vi "IMUOrientOpen.vi"(0 "Op Mode":T6(ring)=enum."NDOF", 1 "Calibrate?":bool, 3 "Stored Cal File":string="BNO055 Cal MC P3 11-28-2015 145653", 5 "Placement":T8(ring)=enum."P3", 9 "I2C Bus":T3=enum."I2C MXP", 11 "Status delay":i32=30, 12 "Alt Adr?":bool, 14 "Flash?":bool) -> (2 "Occupant":u8[](array[numeric]) format="%02x", 4 "IMU Dev Ref":T1={"I2CDevRef"={"DevStatus"={"status"=FALSE, "code"=0, "source"=""}, "Device Address"=0, "Handle"=0, "I2C Bus"=enum."Invalid"}, "Valid Cal File?"=FALSE} {"I2CDevRef"."Device Address" format="%.0x"}, 6 "Cal Status @ Open":T4, 8 "error out":errorcluster, 10 "Fatal Result":bool, 13 "Odd":bool, 15 "Bad Result":bool)   [LabVIEW 2017]
uses:
  <vilib>/Rock Robotics/SystemInterfaces/i2clib/i2c_bus.ctl
  <userlib>/836-Library/Sensor/IMU/Setup State.ctl
  <userlib>/836-Library/Sensor/IMU/ImuDevRef.ctl
  <vilib>/Rock Robotics/WPI/I2C/WPI_I2CDevRef.ctl
panel:
  out "Adr":u8 format="%02x"
  out "Restore Cal ct":i32
  out "Bad ct":i32
  out "SC ct":i32
  out "S":T5
  out "G":T5
  out "A":T5
  out "M":T5
  out "Bad Result":bool
  out "Fusion":bool
  out "Fusion ct":i32
  out "Reset ct":i32
  out "Setup ct":i32
  out "Setup State":T7
  # "Manual Cal\nCalibration Status Indicator"
  # "Diagnostics"
  # "These controls/indicators are non-operational / they are here as example documentation only."
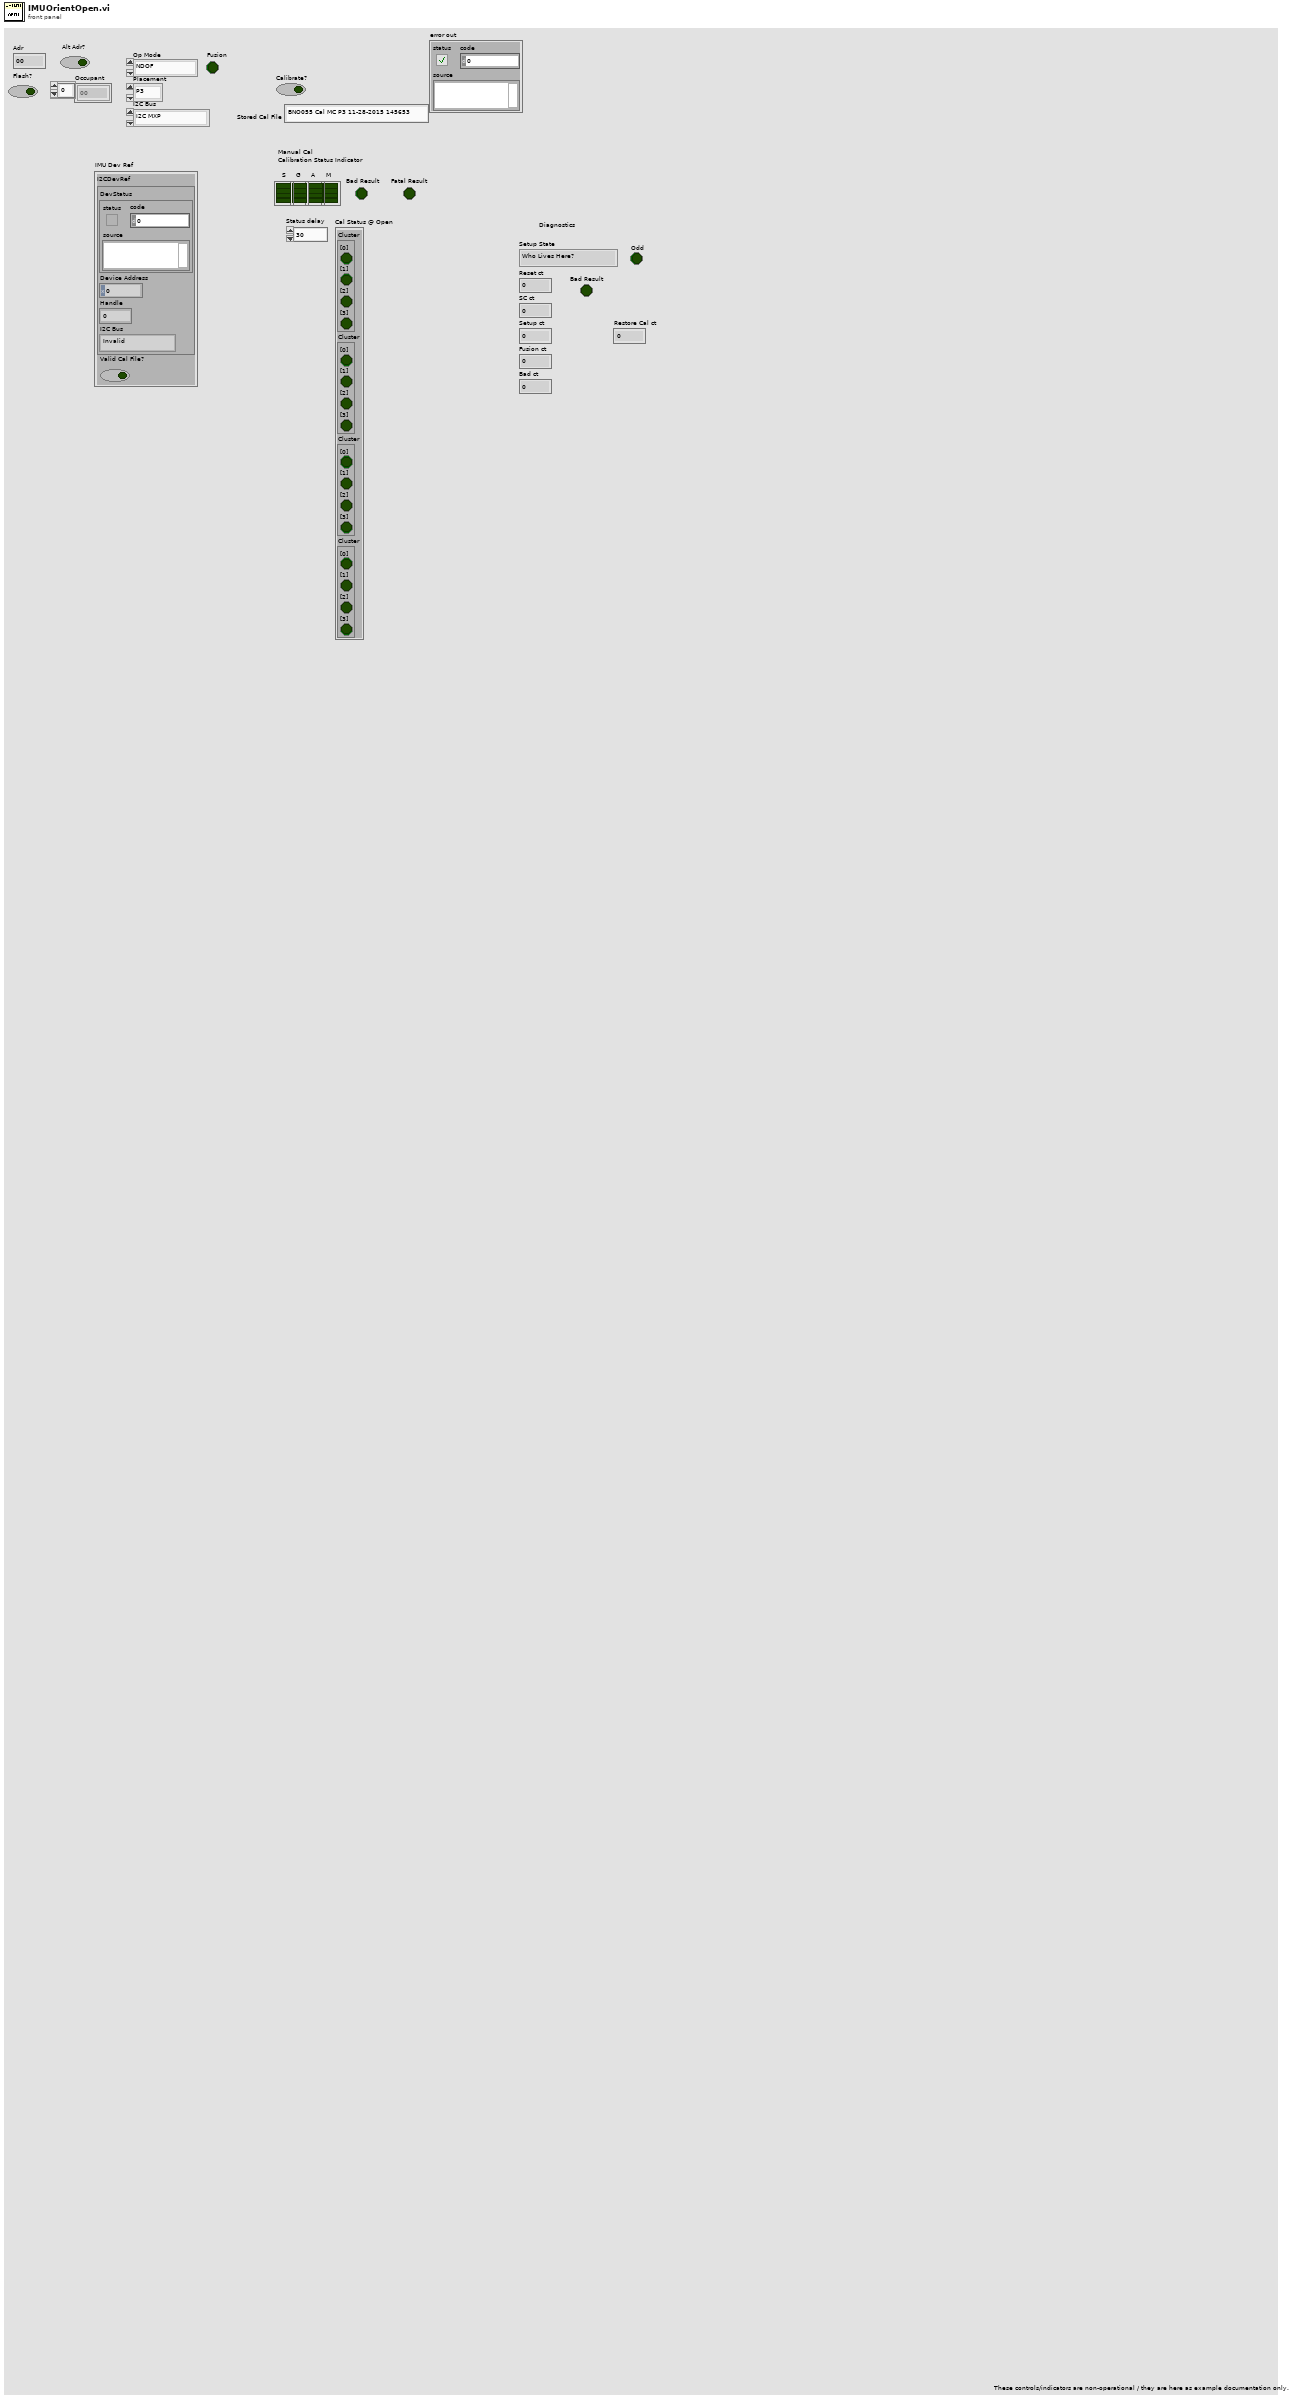
[diagram p1: front panel]
types:
  T1 = typedef "ImuDevRef.ctl" = cluster{"I2CDevRef":T2, "Valid Cal File?":bool}
  T2 = typedef "WPI_I2CDevRef.ctl" = cluster{"DevStatus":errorcluster, "Device Address":u8, "Handle":i32, "I2C Bus":T3}
  T3 = typedef "i2c_bus.ctl" = enum16{"I2C On-Board", "I2C MXP", "Invalid"}
  T4 = cluster{"Cluster":cluster{"[0]":bool, "[1]":bool, "[2]":bool, "[3]":bool}, "Cluster":cluster{"[0]":bool, "[1]":bool, "[2]":bool, "[3]":bool}, "Cluster":cluster{"[0]":bool, "[1]":bool, "[2]":bool, "[3]":bool}, "Cluster":cluster{"[0]":bool, "[1]":bool, "[2]":bool, "[3]":bool}}
  T5 = cluster{"Boolean":bool, "Boolean 2":bool, "Boolean 3":bool, "Boolean 4":bool}
  T6 = enum8{"ConfigMode", "AccOnly", "MagOnly", "GyroOnly", "AccMag", "AccGyro", "MagGyro", "AMG", "IMU", "Compass", "M4G", "NDOF_FMC_OFF", "NDOF"}
  T7 = typedef "Setup State.ctl" = enum16{"Who Lives Here?", "Config Mode", "Page 0", "Reset", "Units, Xtal, & Placement", "Fusion Mode", "Pre Calibration", "Error Check", "Manual Cal", "Save Cal", "Restore Cal", "Cal Status", "Idle"}
  T8 = enum32{"P0", "P1", "P2", "P3", "P4", "P5", "P6", "P7"}
  T9 = enum16{"open", "open or create", "create or replace", "create", "open (read-only)"}
  T10 = enum8{"ConfigMode", "AccOnly", "MagOnly", "GyroOnly", "AccMag", "AccGyro", "MagGyro", "AMG", "IMU", "Compass", "M4G", "NDOF_FMC_OFF", "NDOF"}[]
  T11 = cluster{"[0]":bool, "[1]":bool, "[2]":bool, "[3]":bool}
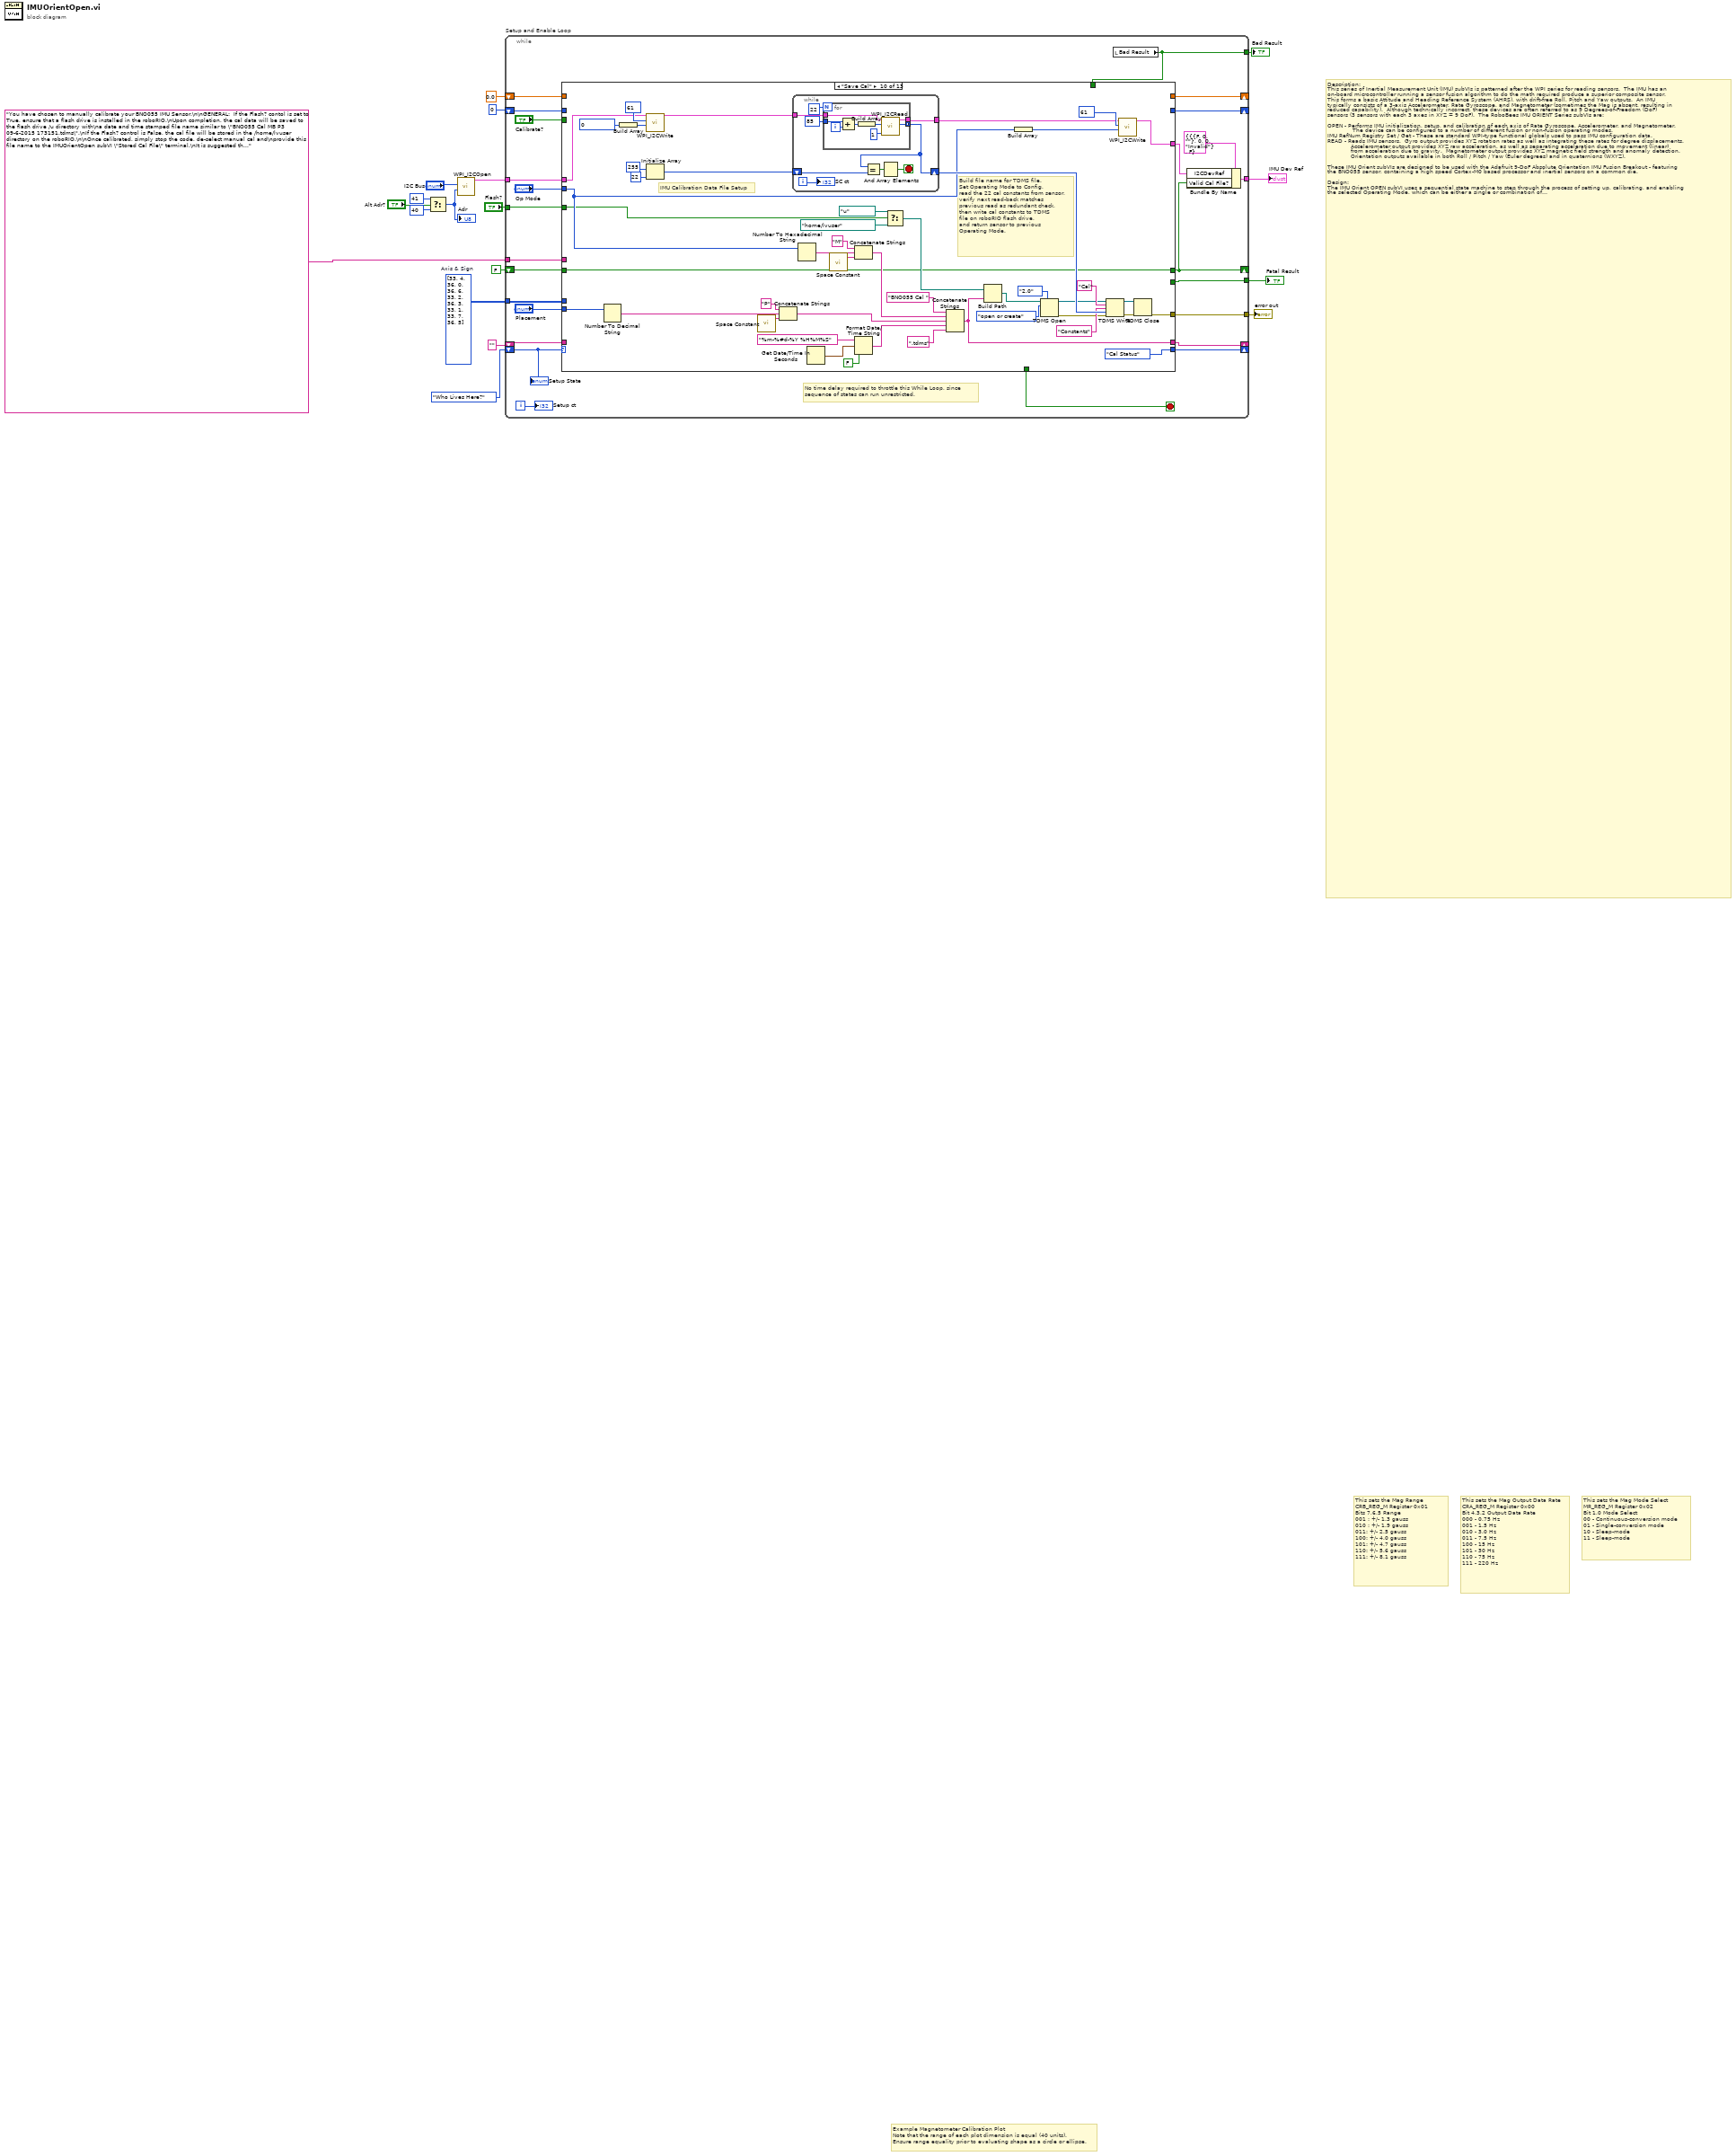
[diagram p0: block diagram]
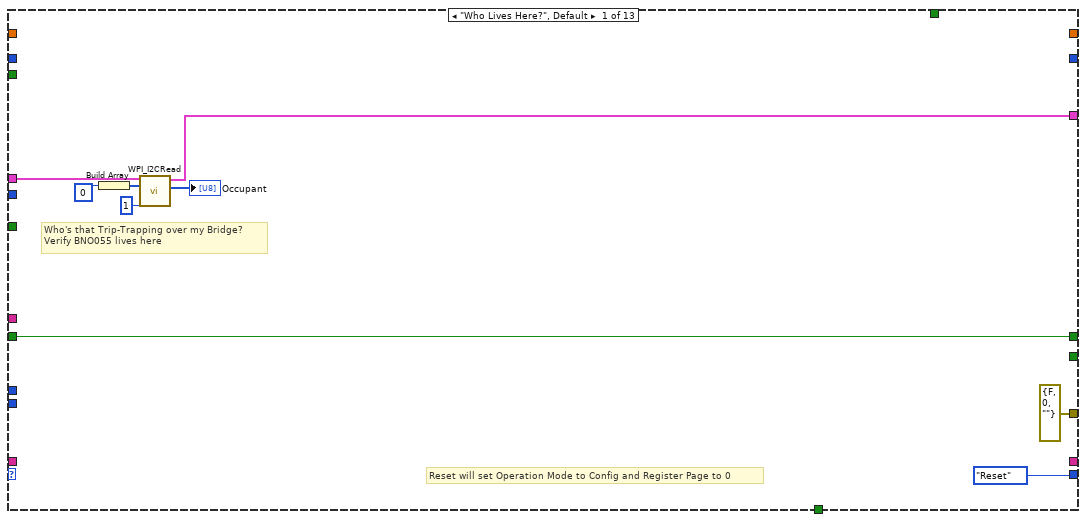
[diagram p2: hidden frame]
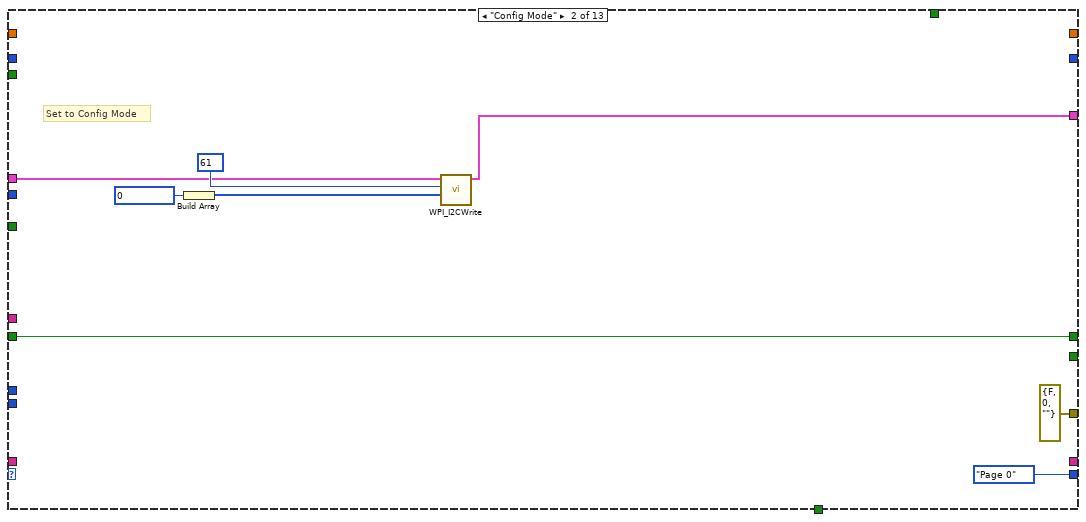
[diagram p3: hidden frame]
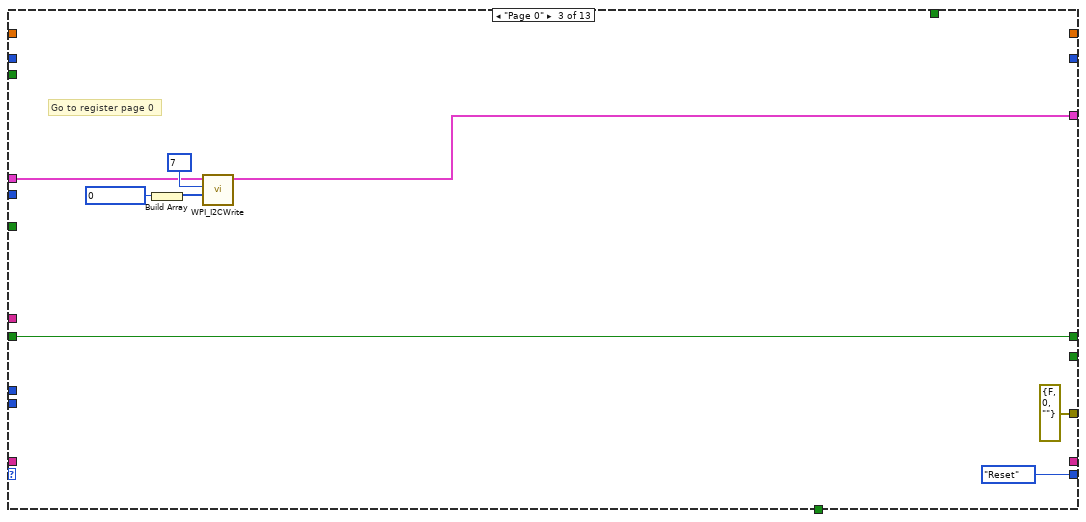
[diagram p4: hidden frame]
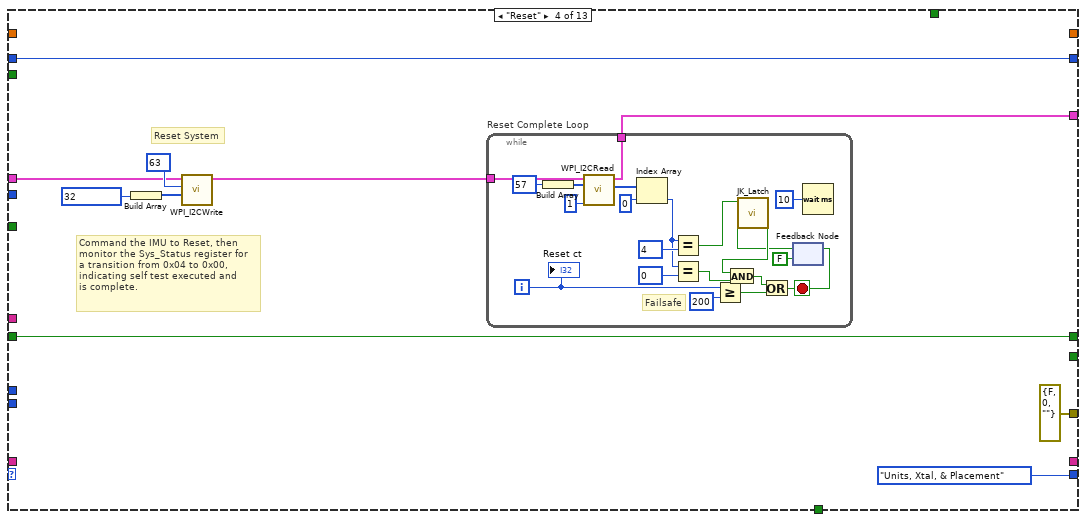
[diagram p5: hidden frame]
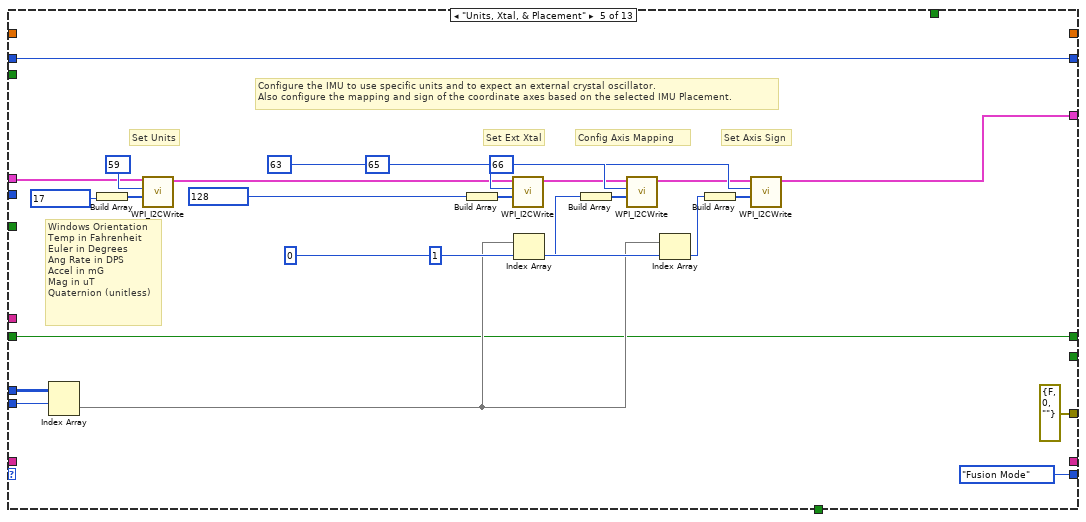
[diagram p6: hidden frame]
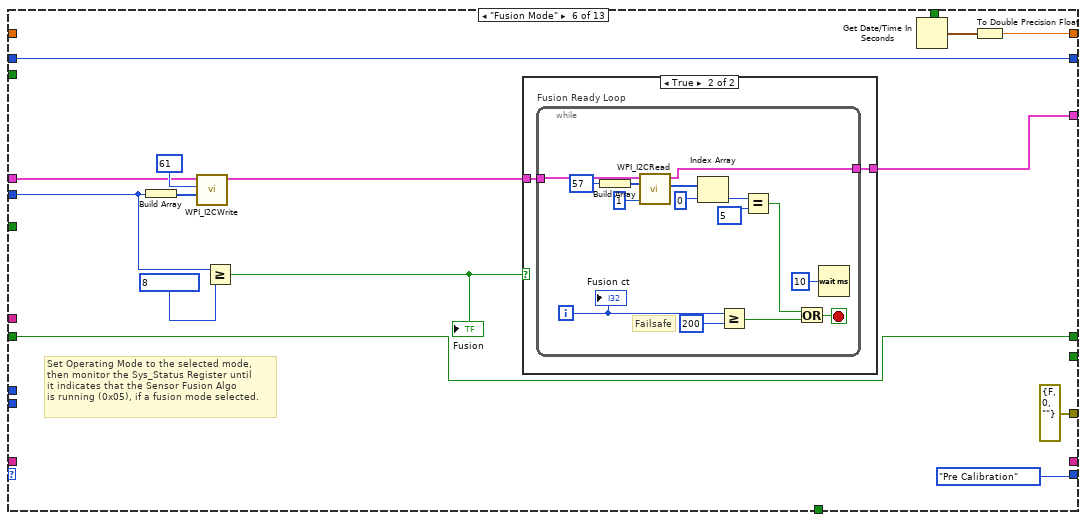
[diagram p7: hidden frame]
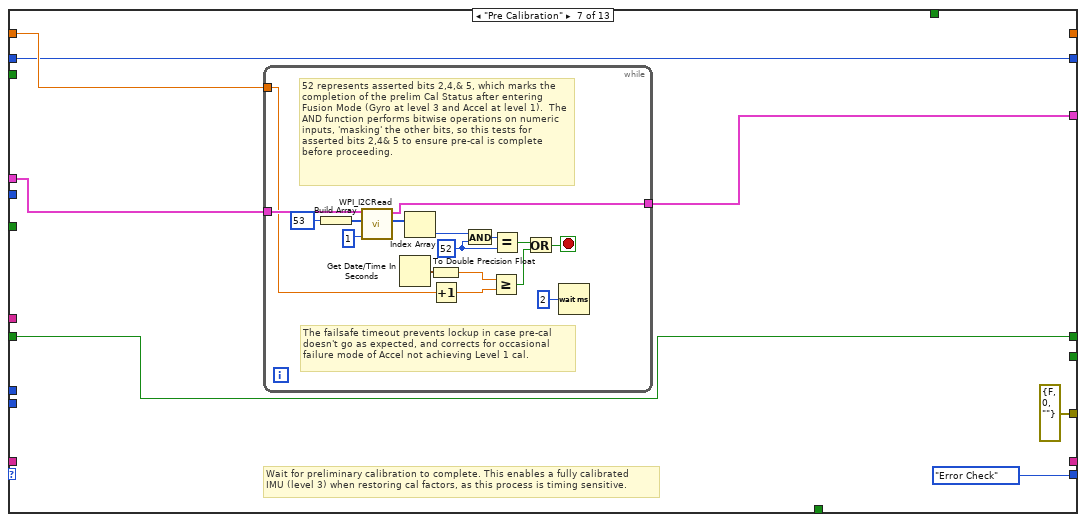
[diagram p9: hidden frame]
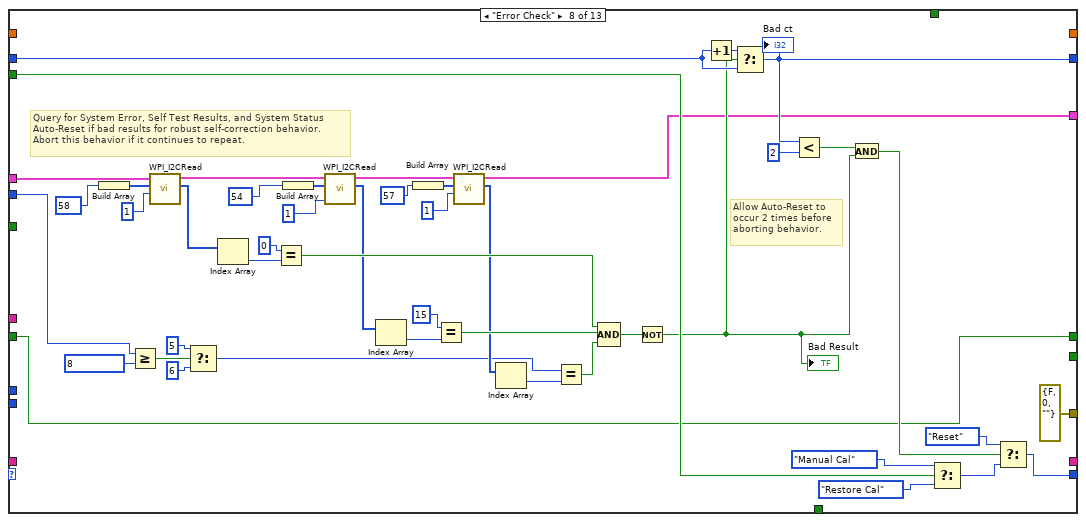
[diagram p10: hidden frame]
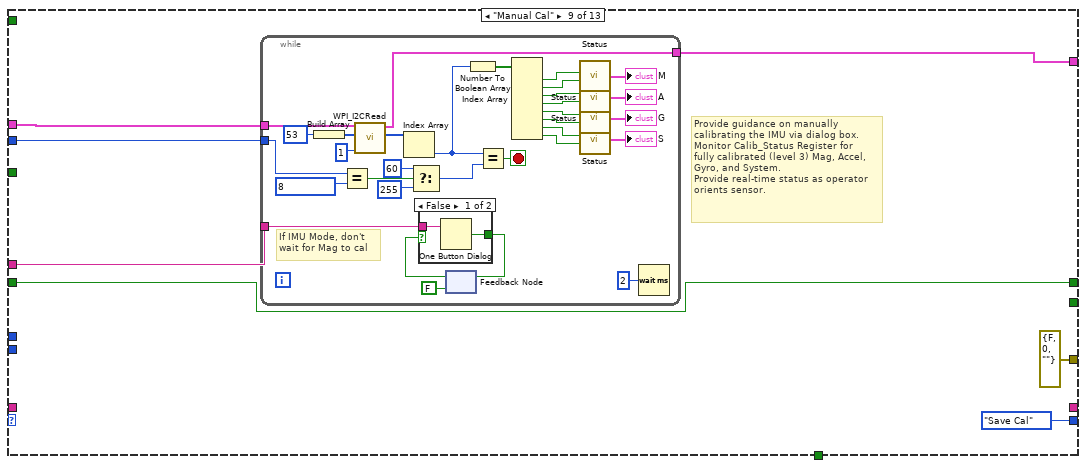
[diagram p11: hidden frame]
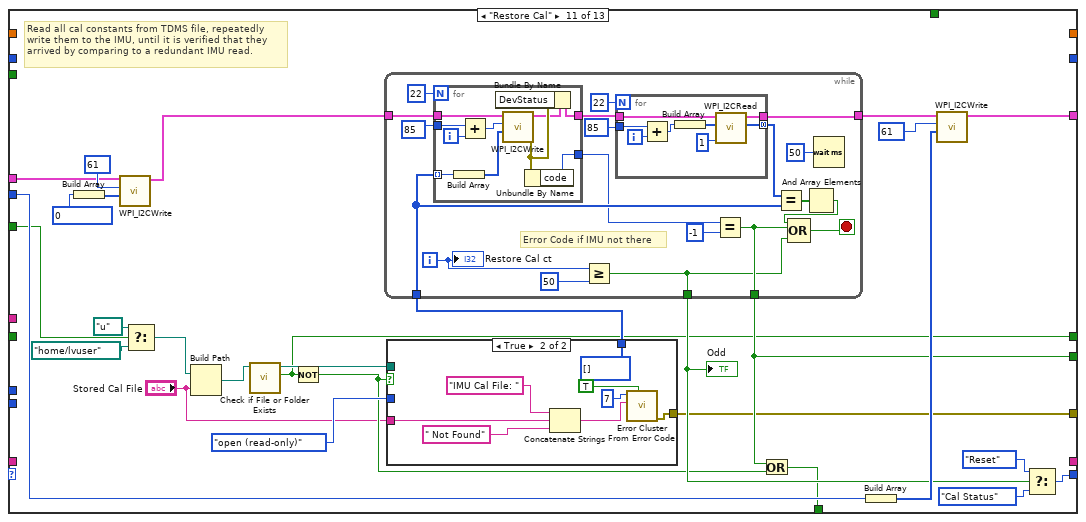
[diagram p13: hidden frame]
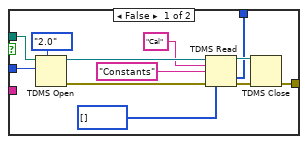
[diagram p14: hidden frame]
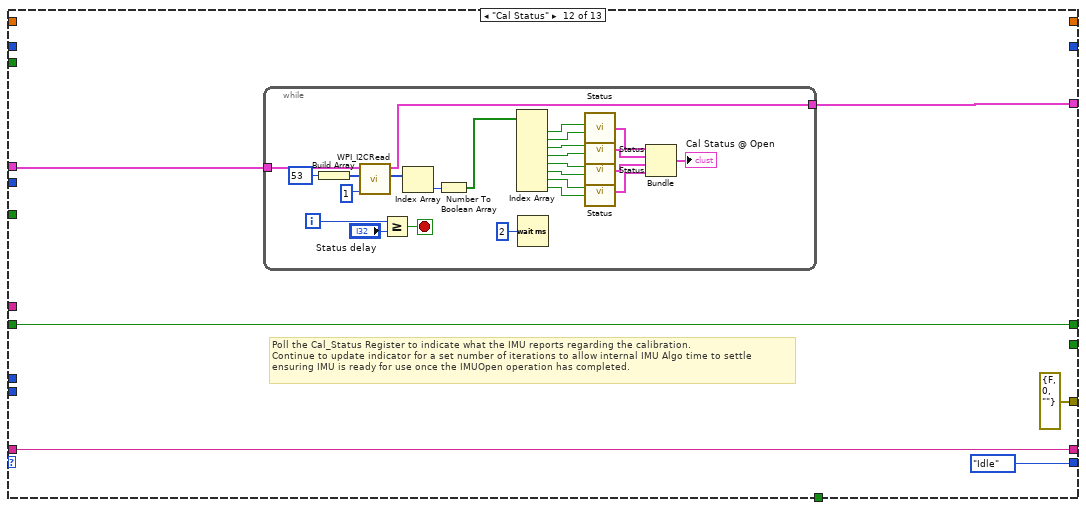
[diagram p15: hidden frame]
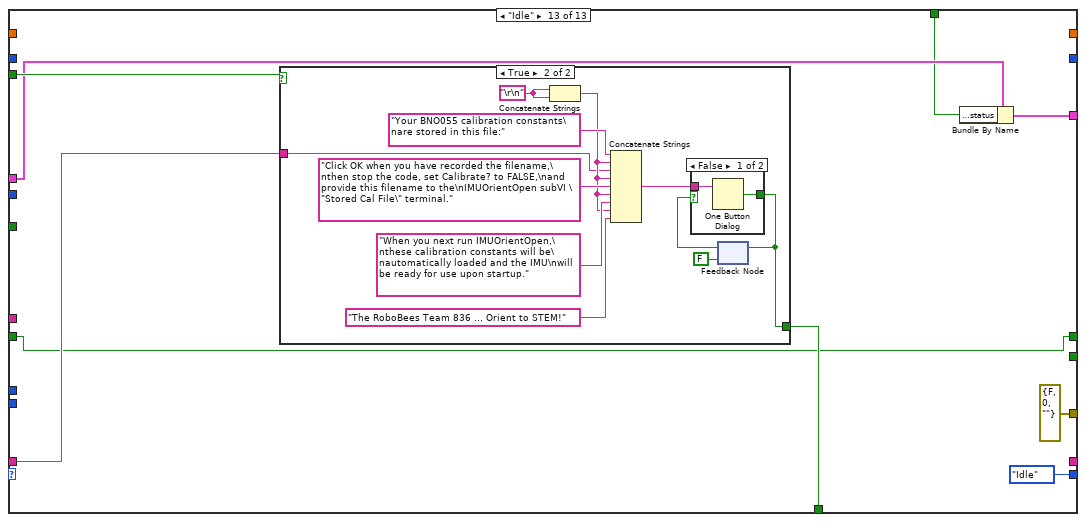
[diagram p16: hidden frame]
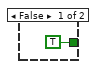
[diagram p17: hidden frame]
diagram:
  w15 = u8[][] [[33, 4], [36, 0], [36, 6], [33, 2], [36, 3], [33, 1], [33, 7], [36, 5]]  # Axis & Sign
  # "Description:\nThis series of Inertial Measurement Unit (IMU) subVIs is patterned after the WPI series for reading sensors.  The IMU has an\non-board microcontroller running a sensor fusion algorithm to do the math required produce a superior composite sensor.\nThis forms a basic Attitude and Heading Reference System (AHRS), with drift-free Roll, Pitch and Yaw outputs.  An IMU\ntypically consists of a 3-axis Accelerometer, Rate Gyroscope, and Magnetometer (sometimes the Mag is absent, resulting in\nreduced capability).  Although technically incorrect, these devices are often referred to as 9 Degrees-of-Freedom (DoF)\nsensors (3 sensors with each 3 axes in XYZ = 9 DoF).  The RoboBees IMU ORIENT Series subVIs are:\n\nOPEN - Performs IMU initialization, setup, and calibration of each axis of Rate Gyroscope, Accelerometer, and Magnetometer.\n              The device can be configured to a number of different fusion or non-fusion operating modes.\nIMU RefNum Registry Set / Get - These are standard WPI-type functional globals used to pass IMU configuration data.\nREAD - Reads IMU sensors.  Gyro output provides XYZ rotation rates as well as integrating these rates for degree displacements.\n             Accelerometer output provides XYZ raw acceleration, as well as separating acceleration due to movement (linear)\n             from acceleration due to gravity.  Magnetometer output provides XYZ magnetic field strength and anomaly detection.\n             Orientation outputs available in both Roll / Pitch / Yaw (Euler degrees) and in quaternions (WXYZ).\n\nThese IMU Orient subVIs are designed to be used with the Adafruit 9-DoF Absolute Orientation IMU Fusion Breakout - featuring\nthe BNO055 sensor, containing a high speed Cortex-M0 based processor and inertial sensors on a common die.\n\nDesign:\nThe IMU Orient OPEN subVI uses a sequential state machine to step through the process of setting up, calibrating, and enabling\nthe selected Operating Mode, which can be either a single or combination of sensors running in a non-fusion mode, or one of\nseveral fusion operating modes.\n\nThe IMU breakout board from Adafruit.com has a single I2C bus for communication.  The sensor I2C Address (in hex) and\ndata sheet for I2C register references are:\n\nI2C Address  -  Data Sheet Reference -\thttps://ae-bst.resource.bosch.com/media/_tech/media/datasheets/BST_BNO055_DS000_14.pdf\n       0x28        -  (Main I2C address, used when Alt Adr? control is False)\n       0x29        -  (Alternate I2C address is used when Alt Adr? control is asserted or True)\n\nNote: The Adafruit website links to an older version of the BNO055 spec sheet (ver 1.2).  The Bosch site will maintain the latest\nversion.  The link above is the latest revision (ver 1.4) as of January 2017 (released June 2016).   This is a highly sophisticated\nsensor, with many control options, so it is recommended that one review the spec sheet to understand all its capabilities.\n\nSome design effort was expended in an attempt to ensure high reliability of operation.  Data transfer between the sensor cal registers\nand the cal file storage location (RIO or flash drive, where cal constants are stored during power down periods) is redundantly verified\nto be successful.  (Testing indicated this to be necessary.)  Upon initialization, if the sensor fails its internal self test, the code will\nattempt to reset the sensor.  This will only occur two times to avoid an infinite loop, which might otherwise prevent a robot from\nexecuting operations code.\n\nCalibration:\nRaw readings from an IMU are not very useful until they are conditioned by carefully determined calibration parameters.  One of\nthe key differences between this IMU and others, such as the one discussed here: \n\n                                                         http://www.chiefdelphi.com/forums/showthread.php?t=131823 \n\nis that this BNO055 contains an integrated microcontroller, running a sensor fusion algorithm, which is designed to constantly\nself-calibrate in real-time, after an initial calibration process has occurred.  So, unlike other IMUs that require interface code, this\nIMU really only requires code to trigger the on-board calibration code.  This makes the code for the sensor READ operations simple,\nand the complex code integration requirement associated only with the sensor OPEN (although one only has to trigger the on-board\ncal process, doing this reliably and providing functionality to store/reload the results still drives code sophistication requirements).\n\nOnce the state machine has initialized the sensor, a user-selected control is referenced to either initiate the sensor's embedded\ncal process or read previously stored calibration constants from a file.  [Note: this vi expects a flash drive to be installed in one\nof the roboRIOs USB ports for cal file storage/retrieval, if the Flash? control is asserted].   A dialog box is used to instruct the user\non the sensor movements required for calibration, and a Calibration Status Indicator is provided on this vi's front panel to provide\nfeedback and track progress.   Once cal is complete, the filename containing the cal constants is displayed.  De-selecting the cal\ncontrol and providing the cal filename to this vi enables the sensor to open in a ready-for-use state.\n\nThe cal filename will contain the Operating Mode, Placement (sensor orientation), and a timestamp to help distinguish one file\nfrom another.  The Op Mode and Placement are included as there is some indication in testing that one should not expect the cal\nto be correct when these parameters differ between cal and use.\n\nVI Properties:\nExecution Reentrancy is set to Pre Allocated Clone Reentrant Execution, enabling multiple Open instances for mutiple IMUs\n\nImplementation:\nIt is recommended that the MXP I2C Interface is used, rather than the On-Board I2C Interface, as the latter can generate glitches from\nLo/Hi byte pairing failures when data is reassembled across paired measurement registers.\n\nA visualization vi is provided to observe orientation change as the sensor is moved.  The vi runs on the My Computer Target,\n(not the roboRIO Target), which means it can only be accessed in debug mode.  There is an issue where Roll exceeding ~45 degrees\ncauses an orientation error.\n \nIt is important to note that while the P/R/Y values are constrained, the Gyro displacement values in X/Y/Z are not.  Gyro deg outputs\nfrom the IMU ORIENT READ subVI will wind (not wrap) - i.e. they will continue to count above/below 360 degrees.  Use the LabVIEW\nQuotient & Remainder (modulus) function to convert these outputs to a wrapping behavior, if desired. \n\nImplementation considerations for IMU Read:\nThis design performs numerical integration off-FPGA for the Digital Gyro (unlike the Analog Gyro subVIs, which typically utilize\nthe FPGA to perform accumulation for superior speed resulting in less integration error).   Testing indicates this off-FPGA\napproach may be adequate for FRC application, however, it is important to ensure the code runs without any timing issues.\nThis is why a Timed Loop is recommended for the IMU Read within Periodic Tasks (executes at a higher priority).  Non-uniformity\nin read iteration is mitigated by design, as each dt is uniquely calculated by time stamping each read event.  This means that while\nsome variation in timing can be tolerated (the occasional late iteration), excessively long durations (periods) between successive\nreads will fail to capture the actual rate profile as it changes resulting in integration error.  \n\nIn short, use a Timed Loop structure to iterate IMU READs, and set the loop period for a relatively fast iteration (<75 ms).  Shorter\nperiods provide improved accuracy of degree displacements, however setting this too short can impact the execution of your\nremaining code (especially when using Timed Loops).  One way of determining an optimized period is to set it while monitoring\nthe \"Finished Late?\" Loop parameter, ensuring this value stays False.   It helps if the CPU Utilization remains low (<75%), which\ncan be monitored with the RT Get CPU Loads subVI (Real Time menu).  Study LabVIEW determinism for additional insight.\n\n----- RoboBees FRC Team 836! -----  You too can conquer inertia!! ... ORIENT on a career in STEM!"
  # "Example Magnetometer Calibration Plot\nNote that the range of each plot dimension is equal (40 units).\nEnsure range equality prior to evaluating shape as a circle or ellipse."
  # "This sets the Mag Mode Select\nMR_REG_M Register 0x02\nBit 1,0 Mode Select\n00 - Continuous-conversion mode \n01 - Single-conversion mode\n10 - Sleep-mode\n11 - Sleep-mode"
  # "This sets the Mag Output Data Rate\nCRA_REG_M Register 0x00\nBit 4,3,2 Output Data Rate\n000 - 0.75 Hz \n001 - 1.5 Hz \n010 - 3.0 Hz\n011 - 7.5 Hz\n100 - 15 Hz\n101 - 30 Hz\n110 - 75 Hz\n111 - 220 Hz"
  # "This sets the Mag Range\nCRB_REG_M Register 0x01\nBits 7,6,5 Range\n001 : +/- 1.3 gauss\n010 : +/- 1.9 gauss\n011: +/- 2.5 gauss\n100: +/- 4.0 gauss\n101: +/- 4.7 gauss\n110: +/- 5.6 gauss\n111: +/- 8.1 gauss"
  n1 = Select(t=u8 41 ("Device Address"), s="Alt Adr?", f=u8 40 ("Device Address")) -> (s? t:f=w6:u8)
  "Adr" <- w6
  n2 = call <vilib>:"WPI_I2COpen.vi"("Device Address"=w6, "I2C Bus"="I2C Bus") -> ("I2CDevRef"=w16:T2)  [unwired: 8 in, 1 out]
  n3 = while "Setup and Enable Loop" {
    tunnel: w16 -> [w37]
    tunnel: "You have chosen to manually calibrate your BNO055 IMU Sensor.\n\nGENERAL:  If the Flash? contol is set to True, ensure that a flash drive is installed in the roboRIO.\nUpon completion, the cal data will be saved to the flash drive /u directory with\na date and time stamped file name similar to \"BNO055 Cal MB P3 09-6-2015 173151.tdms\".\nIf the Flash? control is False, the cal file will be stored in the /home/lvuser directory on the roboRIO.\n\nOnce calibrated, simply stop the code, de-select manual cal and\nprovide this file name to the IMUOrientOpen subVI \"Stored Cal File\" terminal.\nIt is suggested that manual calibration be performed whenever one re-locates\nthe IMU sensor or adds/changes the metallic configuration of the robot.\n\nPREPARATIONS:  If sensor is installed on a robot, ensure sensor is secure.\nThese device movement instructions will then apply to entire robot.\nAs you proceed, monitor the Calibration Status Indicator on the IMUOrientOpen Front Panel.\nCalibration is complete when all indicators are Green.\n\nGYRO CAL:  Allow device to maintain a single stable\nposition to enable Gyro to self-calibrate.\n\nACCELEROMETER CAL:  Place device in 6 different stable\npositions for a few seconds to allow it to calibrate.\nEnsure there is slow movement between 2 stable positions.\nThe 6 stable positions can be in any direction, but ensure the\ndevice is perpendicular to the X,Y & Z axis at least once.\nThis is usually the most difficult device to calibrate.\nIf problematic, try slowing down the movement between positions.\n\nMAGNETOMETER CAL:  Make random movements\nin all 3 axes until Cal Status Indicator is Green.\n\nSYSTEM CAL:  Alternately move device and hold still until\nCal Status Indicator is Green, if necessary. \n\nClick OK when ready to begin." ("message") -> [w42]
    tunnel: w15 -> [w40]
    shift-right: [w35] -> _
    shift-left: 0 -> [w34]
    tunnel: [w26] -> w13
    shift-right: [w33] -> _
    shift-left: 0.0 -> [w32]
    shift-right: [w31] -> _
    shift-left: "" -> [w30]
    shift-right: [w29] -> _
    shift-left: Setup_State."Who Lives Here?" -> [w28]
    tunnel: [w27] -> w9
    tunnel: "Flash?" -> [w25]
    tunnel: [w24] -> w3
    tunnel: [w21] -> w2
    shift-right: [w20] -> _
    shift-left: FALSE ("file or folder exists?") -> [w19]
    i -> [w39]
    stop <- w38 stop-if-true
    # "No time delay required to throttle this While Loop, since sequence of states can run unrestricted."
    n4 = local read "Bad Result"() -> (w26:bool)
    n5 = case shown="\"Save Cal\"" w28 {
      tunnel: [Setup_State."Reset" Setup_State."Page 0" Setup_State."Reset" Setup_State."Units, Xtal, & Placement" Setup_State."Fusion Mode" Setup_State."Pre Calibration" Setup_State."Error Check" w200 Setup_State."Save Cal" Setup_State."Cal Status" w341 Setup_State."Idle" Setup_State."Idle"] -> w29
      tunnel: w37 -> [w49 w56 w65 w75 w117 w137 w164 w216 w234 w309 w354 w423 w453]
      tunnel: "Calibrate?" -> [_ _ _ _ _ _ _ w188 _ _ _ _ w457]
      tunnel: [_ _ _ _ _ w134 _ _ _ _ _ _ _] -> w33
      tunnel: w32 -> [_ _ _ _ _ _ w162 _ _ _ _ _ _]
      tunnel: w42 -> [_ _ _ _ _ _ _ _ w232 _ _ _ _]
      tunnel: "Placement" -> [_ _ _ _ w107 _ _ _ _ w283 _ _ _]
      tunnel: w40 -> [_ _ _ _ w105 _ _ _ _ _ _ _ _]
      tunnel: [_ _ _ _ _ _ _ _ _ w280 _ w421 _] -> w31
      tunnel: [_ _ _ _ _ _ _ _ _ _ w338 _ w456] -> w38
      tunnel: w30 -> [_ _ _ _ _ _ _ _ _ _ _ w421 w455]
      tunnel: "Op Mode" -> [_ _ _ _ _ w130 _ w193 w230 w279 w350 _ _]
      tunnel: [_ _ _ w72 w103 w129 w161 w190 _ _ _ _ _] -> w35
      tunnel: w34 -> [_ _ _ w72 w103 w129 w161 w191 _ _ _ _ _]
      tunnel: [_ _ _ _ _ _ _ _ _ _ w339 _ _] -> w27
      tunnel: [w46 w55 w63 w71 w102 w128 w160 w184 w231 w278 w349 w420 w452] -> w22
      tunnel: w26 -> [_ _ _ _ _ _ _ _ _ _ _ _ w451]
      tunnel: w25 -> [_ _ _ _ _ _ _ _ _ w274 w346 _ _]
      tunnel: [errorcluster {"status"=FALSE, "code"=0, "source"=""} ("error out") errorcluster {"status"=FALSE, "code"=0, "source"=""} ("error out") errorcluster {"status"=FALSE, "code"=0, "source"=""} ("error out") errorcluster {"status"=FALSE, "code"=0, "source"=""} ("error out") errorcluster {"status"=FALSE, "code"=0, "source"=""} ("error out") errorcluster {"status"=FALSE, "code"=0, "source"=""} ("error out") errorcluster {"status"=FALSE, "code"=0, "source"=""} ("error out") errorcluster {"status"=FALSE, "code"=0, "source"=""} ("error out") errorcluster {"status"=FALSE, "code"=0, "source"=""} ("error out") w273 w334 errorcluster {"status"=FALSE, "code"=0, "source"=""} ("error out") errorcluster {"status"=FALSE, "code"=0, "source"=""} ("error out")] -> w24
      tunnel: [w44 w53 w61 w69 w100 w126 w158 w182 w228 w270 w333 w418 w449] -> w20
      tunnel: w19 -> [w44 w53 w61 w69 w100 w126 w158 w182 w228 w270 _ w418 w449]
      frame "Who Lives Here?", Default {
        # "Reset will set Operation Mode to Config and Register Page to 0"
        # "Who's that Trip-Trapping over my Bridge?\nVerify BNO055 lives here"
        n6 = Build Array(u8 0 ("Data To Send")) -> (w52:u8[])
        n7 = call <vilib>:"WPI_I2CRead.vi"("I2CBytesToRead"=u8 1, "I2CRegister"=w52, "I2CDevRef"=w49) -> ("Data Out"=→"Occupant":u8[], "I2CDevRef"=w46:T2)  [unwired: 6 in, 1 out]
      }
      frame "Config Mode" {
        # "Set to Config Mode"
        n8 = Build Array(u8 0 ("I2CRegister")) -> (w60:u8[])
        n9 = call <vilib>:"WPI_I2CWrite.vi"("I2CDataToSend"=w60, "I2CRegister"=u8 61 ("Data To Send hex 2"), "I2CDevRef"=w56) -> ("I2CDevRef"=w55:T2)  [unwired: 7 in, 1 out]
      }
      frame "Page 0" {
        # "Go to register page 0"
        n10 = Build Array(u8 0 ("I2CRegister")) -> (w68:u8[])
        n11 = call <vilib>:"WPI_I2CWrite.vi"("I2CDataToSend"=w68, "I2CRegister"=u8 7 ("Data To Send hex 2"), "I2CDevRef"=w65) -> ("I2CDevRef"=w63:T2)  [unwired: 7 in, 1 out]
      }
      frame "Reset" {
        # "Command the IMU to Reset, then\nmonitor the Sys_Status register for\na transition from 0x04 to 0x00,\nindicating self test executed and\nis complete."
        # "Reset System"
        n12 = Build Array(u8 32 ("I2CRegister")) -> (w78:u8[])
        n13 = call <vilib>:"WPI_I2CWrite.vi"("I2CDataToSend"=w78, "I2CRegister"=u8 63 ("Data To Send hex 2"), "I2CDevRef"=w75) -> ("I2CDevRef"=w73:T2)  [unwired: 7 in, 1 out]
        n14 = while "Reset Complete Loop" {
          tunnel: w73 -> [w94]
          tunnel: [w79] -> w71
          i -> [w82]
          stop <- w84 stop-if-true
          # "Failsafe"
          n15 = Build Array(u8 57 ("Data To Send")) -> (w97:u8[])
          n16 = call <vilib>:"WPI_I2CRead.vi"("I2CBytesToRead"=u8 1, "I2CRegister"=w97, "I2CDevRef"=w94) -> ("Data Out"=w96:u8[], "I2CDevRef"=w79:T2)  [unwired: 6 in, 1 out]
          n17 = Index Array(array=w96, index=0 ("disabled index (col)")) -> (element=w83:u8)
          n18 = Equal?(x=w83, y=u8 4 ("I2CBytesToRead")) -> (x = y?=w89:bool)
          n19 = Equal?(x=w83, y=u8 0 ("I2CBytesToRead")) -> (x = y?=w88:bool)
          n20 = Greater Or Equal?(x=w82, y=200) -> (x >= y?=w86:bool)
          n21 = feedback #1(FALSE) -> (w81:bool)
          n22 = call <userlib>:"JK_Latch.vi"("Reset"=w81, "Set"=w89) -> ("Q"=w90:bool)  [unwired: 5 in]
          n23 = And(x=w90, y=w88) -> (x .and. y?=w87:bool)
          n24 = Or(x=w87, y=w86) -> (x .or. y?=w84:bool)
          n25 = feedback-in #1(w84) -> ()
          n26 = Wait (ms)(milliseconds to wait=u32 10) -> ()  [unwired: 1 out]
          "Reset ct" <- w82
        }
      }
      frame "Units, Xtal, & Placement" {
        # "Configure the IMU to use specific units and to expect an external crystal oscillator.\nAlso configure the mapping and sign of the coordinate axes based on the selected IMU Placement."
        # "Set Axis Sign"
        # "Config Axis Mapping"
        # "Set Ext Xtal"
        # "Windows Orientation\nTemp in Fahrenheit\nEuler in Degrees\nAng Rate in DPS\nAccel in mG\nMag in uT\nQuaternion (unitless)"
        # "Set Units"
        n27 = Index Array(array=w105, index (row)=w107) -> (element=w108:u8[])  [unwired: 1 in]
        n28 = Build Array(u8 17 ("I2CRegister")) -> (w125:u8[])
        n29 = call <vilib>:"WPI_I2CWrite.vi"("I2CDataToSend"=w125, "I2CRegister"=u8 59 ("Data To Send hex 2"), "I2CDevRef"=w117) -> ("I2CDevRef"=w119:T2)  [unwired: 7 in, 1 out]
        n30 = Build Array(u8 128 ("I2CRegister")) -> (w124:u8[])
        n31 = call <vilib>:"WPI_I2CWrite.vi"("I2CDataToSend"=w124, "I2CRegister"=u8 63 ("Data To Send hex 2"), "I2CDevRef"=w119) -> ("I2CDevRef"=w114:T2)  [unwired: 7 in, 1 out]
        n32 = Index Array(array=w108, index=0) -> (element=w106:u8)
        n33 = Build Array(w106) -> (w115:u8[])
        n34 = call <vilib>:"WPI_I2CWrite.vi"("I2CDataToSend"=w115, "I2CRegister"=u8 65 ("Data To Send hex 2"), "I2CDevRef"=w114) -> ("I2CDevRef"=w111:T2)  [unwired: 7 in, 1 out]
        n35 = Index Array(array=w108, index=1) -> (element=w104:u8)
        n36 = Build Array(w104) -> (w113:u8[])
        n37 = call <vilib>:"WPI_I2CWrite.vi"("I2CDataToSend"=w113, "I2CRegister"=u8 66 ("Data To Send hex 2"), "I2CDevRef"=w111) -> ("I2CDevRef"=w102:T2)  [unwired: 7 in, 1 out]
      }
      frame "Fusion Mode" {
        # "Set Operating Mode to the selected mode,\nthen monitor the Sys_Status Register until\nit indicates that the Sensor Fusion Algo\nis running (0x05), if a fusion mode selected."
        n38 = Build Array(w130) -> (w139:T10)
        n39 = call <vilib>:"WPI_I2CWrite.vi"("I2CDataToSend"=w139, "I2CRegister"=u8 61 ("Data To Send hex 2"), "I2CDevRef"=w137) -> ("I2CDevRef"=w136:T2)  [unwired: 7 in, 1 out]
        n40 = Greater Or Equal?(x=w130, y=u8 8 ("I2CRegister")) -> (x >= y?=w132:bool)
        "Fusion" <- w132
        n41 = case shown="True" w132 {
          tunnel: w136 -> [w140 w142]
          tunnel: [w140 w141] -> w128
          frame False {
          }
          frame True {
            n42 = while "Fusion Ready Loop" {
              tunnel: w142 -> [w152]
              tunnel: [w143] -> w141
              i -> [w147]
              stop <- w151 stop-if-true
              # "Failsafe"
              n43 = Build Array(u8 57 ("Data To Send")) -> (w155:u8[])
              n44 = call <vilib>:"WPI_I2CRead.vi"("I2CBytesToRead"=u8 1, "I2CRegister"=w155, "I2CDevRef"=w152) -> ("Data Out"=w154:u8[], "I2CDevRef"=w143:T2)  [unwired: 6 in, 1 out]
              n45 = Index Array(array=w154, index=0 ("disabled index (col)")) -> (element=w144:u8)
              n46 = Greater Or Equal?(x=w147, y=200) -> (x >= y?=w148:bool)
              n47 = Equal?(x=w144, y=u8 5 ("I2CBytesToRead")) -> (x = y?=w150:bool)
              n48 = Or(x=w150, y=w148) -> (x .or. y?=w151:bool)
              n49 = Wait (ms)(milliseconds to wait=u32 10) -> ()  [unwired: 1 out]
              "Fusion ct" <- w147
            }
          }
        }
        n50 = Get Date/Time In Seconds() -> (seconds since 1Jan1904=w135:timestamp)
        n51 = To Double Precision Float(number=w135) -> (double precision float=w134:dbl)
      }
      frame "Pre Calibration" {
        # "Wait for preliminary calibration to complete. This enables a fully calibrated\nIMU (level 3) when restoring cal factors, as this process is timing sensitive."
        n52 = while {
          tunnel: w164 -> [w177]
          tunnel: w162 -> [w167]
          tunnel: [w165] -> w160
          stop <- w172 stop-if-true
          w173 = u8 52 ("y")
          # "The failsafe timeout prevents lockup in case pre-cal\ndoesn't go as expected, and corrects for occasional\nfailure mode of Accel not achieving Level 1 cal."
          # "52 represents asserted bits 2,4,& 5, which marks the completion of the prelim Cal Status after entering Fusion Mode (Gyro at level 3 and Accel at level 1).  The AND function performs bitwise operations on numeric inputs, 'masking' the other bits, so this tests for asserted bits 2,4& 5 to ensure pre-cal is complete before proceeding."
          n53 = Build Array(u8 53 ("Data To Send")) -> (w181:u8[])
          n54 = call <vilib>:"WPI_I2CRead.vi"("I2CBytesToRead"=u8 1, "I2CRegister"=w181, "I2CDevRef"=w177) -> ("Data Out"=w178:u8[], "I2CDevRef"=w165:T2)  [unwired: 6 in, 1 out]
          n55 = Get Date/Time In Seconds() -> (seconds since 1Jan1904=w171:timestamp)
          n56 = Index Array(array=w178) -> (element=w174:u8)  [unwired: 1 in]
          n57 = To Double Precision Float(number=w171) -> (double precision float=w168:dbl)
          n58 = Increment(x=w167) -> (x+1=w166:dbl)
          n59 = And(x=w174, y=w173) -> (x .and. y?=w175:u8)
          n60 = Greater Or Equal?(x=w168, y=w166) -> (x >= y?=w169:bool)
          n61 = Equal?(x=w175, y=w173) -> (x = y?=w170:bool)
          n62 = Or(x=w170, y=w169) -> (x .or. y?=w172:bool)
          n63 = Wait (ms)(milliseconds to wait=u32 2 ("pre-cal wait")) -> ()  [unwired: 1 out]
        }
      }
      frame "Error Check" {
        # "Allow Auto-Reset to\noccur 2 times before\naborting behavior."
        # "Query for System Error, Self Test Results, and System Status\nAuto-Reset if bad results for robust self-correction behavior.\nAbort this behavior if it continues to repeat."
        n64 = Build Array(u8 58 ("Data To Send")) -> (w225:u8[])
        n65 = Greater Or Equal?(x=w193, y=u8 8 ("I2CRegister")) -> (x >= y?=w198:bool)
        n66 = call <vilib>:"WPI_I2CRead.vi"("I2CBytesToRead"=u8 1, "I2CRegister"=w225, "I2CDevRef"=w216) -> ("Data Out"=w207:u8[], "I2CDevRef"=w218:T2)  [unwired: 6 in, 1 out]
        n67 = Select(t=u8 5 ("x"), s=w198, f=u8 6 ("x")) -> (s? t:f=w195:u8)
        n68 = Index Array(array=w207) -> (element=w208:u8)  [unwired: 1 in]
        n69 = Equal?(x=u8 0, y=w208) -> (x = y?=w212:bool)
        n70 = Build Array(u8 54 ("Data To Send")) -> (w224:u8[])
        n71 = call <vilib>:"WPI_I2CRead.vi"("I2CBytesToRead"=u8 1, "I2CRegister"=w224, "I2CDevRef"=w218) -> ("Data Out"=w206:u8[], "I2CDevRef"=w217:T2)  [unwired: 6 in, 1 out]
        n72 = Index Array(array=w206) -> (element=w209:u8)  [unwired: 1 in]
        n73 = Build Array(u8 57 ("Data To Send")) -> (w219:u8[])
        n74 = Equal?(x=u8 15, y=w209) -> (x = y?=w213:bool)
        n75 = call <vilib>:"WPI_I2CRead.vi"("I2CBytesToRead"=u8 1, "I2CRegister"=w219, "I2CDevRef"=w217) -> ("Data Out"=w205:u8[], "I2CDevRef"=w184:T2)  [unwired: 6 in, 1 out]
        n76 = Index Array(array=w205) -> (element=w211:u8)  [unwired: 1 in]
        n77 = Equal?(x=w195, y=w211) -> (x = y?=w214:bool)
        n78 = Compound Arithmetic op=AND(w212, w213, w214) -> (w215:bool)
        n79 = Not(x=w215) -> (.not. x?=w186:bool)
        "Bad Result" <- w186
        n80 = Increment(x=w191) -> (x+1=w192:i32)
        n81 = Select(t=w192, s=w186, f=w191) -> (s? t:f=w190:i32)
        "Bad ct" <- w190
        n82 = Less?(x=w190, y=2) -> (x < y?=w185:bool)
        n83 = And(x=w185, y=w186) -> (x .and. y?=w187:bool)
        n84 = Select(t=Setup_State."Manual Cal", s=w188, f=Setup_State."Restore Cal") -> (s? t:f=w201:T7)
        n85 = Select(t=Setup_State."Reset", s=w187, f=w201) -> (s? t:f=w200:T7)
      }
      frame "Manual Cal" {
        # "Provide guidance on manually\ncalibrating the IMU via dialog box.\nMonitor Calib_Status Register for\nfully calibrated (level 3) Mag, Accel,\nGyro, and System. \nProvide real-time status as operator\norients sensor."
        n86 = while {
          tunnel: w234 -> [w263]
          tunnel: w232 -> [w248]
          tunnel: [w246] -> w231
          tunnel: w230 -> [w244]
          stop <- w247 stop-if-true
          # "If IMU Mode, don't\nwait for Mag to cal"
          n87 = Build Array(u8 53 ("Data To Send")) -> (w266:u8[])
          n88 = Equal?(x=w244, y=u8 8 ("I2CRegister")) -> (x = y?=w240:bool)
          n89 = call <vilib>:"WPI_I2CRead.vi"("I2CBytesToRead"=u8 1, "I2CRegister"=w266, "I2CDevRef"=w263) -> ("Data Out"=w264:u8[], "I2CDevRef"=w246:T2)  [unwired: 6 in, 1 out]
          n90 = Index Array(array=w264) -> (element=w252:u8)  [unwired: 1 in]
          n91 = Select(t=u8 60 ("y"), s=w240, f=u8 255 ("y")) -> (s? t:f=w239:u8)
          n92 = feedback #2(FALSE ("true")) -> (w250:bool)
          n93 = case shown="False" w250 {
            selector: w250 -> [_ w269]
            tunnel: [w268 w269] -> w251
            tunnel: w248 -> [w267 _]
            frame False {
              n94 = One Button Dialog(message=w267) -> (true=w268:bool)  [unwired: 1 in]
            }
            frame True {
            }
          }
          n95 = feedback-in #2(w251) -> ()
          n96 = Number To Boolean Array(number=w252) -> (Boolean array=w253:bool[])
          n97 = Equal?(x=w252, y=w239) -> (x = y?=w247:bool)
          n98 = Index Array(array=w253) -> (element #1=w261:bool, element #2=w260:bool, element #3=w259:bool, element #4=w258:bool, element #5=w257:bool, element #6=w256:bool, element #7=w255:bool, element #8=w254:bool)  [unwired: 8 in]
          n99 = call <userlib>:"Status.vi"("Big"=w260, "Little"=w261) -> ("Cluster"=→"M":T11)  [unwired: 2 in]
          n100 = call <userlib>:"Status.vi"("Big"=w258, "Little"=w259) -> ("Cluster"=→"A":T11)  [unwired: 2 in]
          n101 = call <userlib>:"Status.vi"("Big"=w256, "Little"=w257) -> ("Cluster"=→"G":T11)  [unwired: 2 in]
          n102 = call <userlib>:"Status.vi"("Big"=w254, "Little"=w255) -> ("Cluster"=→"S":T11)  [unwired: 2 in]
          n103 = Wait (ms)(milliseconds to wait=u32 2 ("pre-cal wait")) -> ()  [unwired: 1 out]
        }
      }
      frame "Save Cal" {
        # "Build file name for TDMS file.\nSet Operating Mode to Config,\nread the 22 cal constants from sensor,\nverify next read-back matches\nprevious read as redundant check,\nthen write cal constants to TDMS\nfile on roboRIO flash drive,\nand return sensor to previous\nOperating Mode."
        # "IMU Calibration Data File Setup"
        n104 = Number To Decimal String(number=w283) -> (decimal integer string=w290:string)  [unwired: 1 in]
        n105 = Build Array(u8 0 ("I2CRegister")) -> (w313:u8[])
        n106 = call <vilib>:"WPI_I2CWrite.vi"("I2CDataToSend"=w313, "I2CRegister"=u8 61 ("Data To Send hex 2"), "I2CDevRef"=w309) -> ("I2CDevRef"=w308:T2)  [unwired: 7 in, 1 out]
        n107 = Initialize Array(u8 255, 22 ("dimension size")) -> (w301:u8[])
        n108 = call <vilib>:"Space Constant.vi"() -> ("String"=w289:string)
        n109 = Concatenate Strings("P" ("string"), w290, w289) -> (w284:string)
        n110 = while {
          tunnel: w308 -> [w319]
          shift-right: [w316] -> w305
          shift-left: w301 -> [w322]
          tunnel: [w320] -> w306
          i -> [w318]
          stop <- w321 stop-if-true
          n111 = for {
            N: 22 -> [_]
            tunnel: u8 85 ("Data To Send 2") -> [w329]
            tunnel: [w327] -> w316 mode=concatenating
            tunnel: w319 -> [w326]
            tunnel: [w325] -> w320
            i -> [w328]
            n112 = Add(x=w329, y=w328) -> (x+y=w330:i32)
            n113 = Build Array(w330) -> (w331:i32[])
            n114 = call <vilib>:"WPI_I2CRead.vi"("I2CBytesToRead"=u8 1, "I2CRegister"=w331, "I2CDevRef"=w326) -> ("Data Out"=w327:u8[], "I2CDevRef"=w325:T2)  [unwired: 6 in, 1 out]
          }
          n115 = Equal?(x=w316, y=w322) -> (x = y?=w317:bool[])
          n116 = And Array Elements(Boolean array=w317) -> (logical AND=w321:bool)
          "SC ct" <- w318
        }
        n117 = Number To Hexadecimal String(2:w279) -> (0:w286:string)  [unwired: 1 in]
        n118 = Get Date/Time In Seconds() -> (seconds since 1Jan1904=w294:timestamp)
        n119 = call <vilib>:"Space Constant.vi"() -> ("String"=w288:string)
        n120 = Concatenate Strings("M" ("string"), w286, w288) -> (w285:string)
        n121 = Format Date/Time String(time format string (%c)="%m-%#d-%Y %H%M%S", seconds (now)=w294, UTC format=FALSE) -> (date/time string=w292:string)
        n122 = Select(t=path "u:/" ("file path (dialog if empty)"), s=w274, f=path "/home/lvuser" ("file path (dialog if empty)")) -> (s? t:f=w275:path)
        n123 = Concatenate Strings("BNO055 Cal " ("string"), w285, w284, w292, ".tdms" ("string")) -> (w280:string)
        n124 = Build Path(base path=w275, name or relative path=w280) -> (appended path=w298:path)
        n125 = Build Array(w279) -> (w315:T10)
        n126 = TDMS Open(7:enum16{"1.0", "2.0"}."2.0" ("file format version (2.0)"), 10:T9."open or create" ("operation (0:open)"), 11:w298) -> (0:w271:errorcluster, 3:w282:refnum<k34>)  [unwired: 4 in]
        n127 = TDMS Write(0:w282, 5:"Cal" ("group name in (Untitled)"), 7:"Constants" ("channel name(s) in"), 9:w305, 11:w271) -> (4:w281:refnum<k34>, 15:w272:errorcluster)  [unwired: 1 in, 2 out]
        n128 = call <vilib>:"WPI_I2CWrite.vi"("I2CDataToSend"=w315, "I2CRegister"=u8 61 ("Data To Send hex 2"), "I2CDevRef"=w306) -> ("I2CDevRef"=w278:T2)  [unwired: 7 in, 1 out]
        n129 = TDMS Close(8:w272, 11:w281) -> (0:w273:errorcluster)  [unwired: 1 out]
      }
      frame "Restore Cal" {
        # "Read all cal constants from TDMS file, repeatedly\nwrite them to the IMU, until it is verified that they\narrived by comparing to a redundant IMU read."
        n130 = Build Array(u8 0 ("I2CRegister")) -> (w356:u8[])
        n131 = call <vilib>:"WPI_I2CWrite.vi"("I2CDataToSend"=w356, "I2CRegister"=u8 61 ("Data To Send hex 2"), "I2CDevRef"=w354) -> ("I2CDevRef"=w353:T2)  [unwired: 7 in, 1 out]
        n132 = Select(t=path "u:/" ("file path (dialog if empty)"), s=w346, f=path "/home/lvuser" ("file path (dialog if empty)")) -> (s? t:f=w345:path)
        n133 = Build Path(base path=w345, name or relative path="Stored Cal File") -> (appended path=w340:path)
        n134 = call <vilib>:"Check if File or Folder Exists.vi"("path"=w340) -> ("file or folder exists?"=w333:bool, "dup path"=w335:path)  [unwired: 8 in, 1 out]
        n135 = Not(x=w333) -> (.not. x?=w337:bool)
        n136 = case shown="True" w337 {
          tunnel: T9."open (read-only)" ("operation (0:open)") -> [w369 _]
          tunnel: [w365 u8[] []] -> w352
          tunnel: [w364 w377] -> w334
          tunnel: "Stored Cal File" -> [_ w374]
          tunnel: w335 -> [w361 _]
          frame False {
            n137 = TDMS Open(7:enum16{"1.0", "2.0"}."2.0" ("file format version (2.0)"), 10:w369, 11:w361) -> (0:w362:errorcluster, 3:w371:refnum<k34>)  [unwired: 4 in]
            n138 = TDMS Read(0:w371, 5:"Cal" ("group name in (Untitled)"), 7:"Constants" ("channel name(s) in"), 11:w362, 12:u8[] []) -> (4:w372:refnum<k34>, 10:w365:u8[], 15:w363:errorcluster)  [unwired: 3 in, 3 out]
            n139 = TDMS Close(8:w363, 11:w372) -> (0:w364:errorcluster)  [unwired: 1 out]
          }
          frame True {
            n140 = Concatenate Strings("IMU Cal File: " ("string"), w374, " Not Found" ("string")) -> (w376:string)
            n141 = call <vilib>:"Error Cluster From Error Code.vi"("show call chain? (False)"=TRUE, "error message (\"\")"=w376, "error code (0)"=7) -> ("error out"=w377:errorcluster)  [unwired: 6 in]
          }
        }
        n142 = while {
          tunnel: w352 -> [w392]
          tunnel: w353 -> [w397]
          tunnel: [w391] -> w351
          tunnel: [w384] -> w339
          tunnel: [w381] -> w342
          i -> [w383]
          stop <- w387 stop-if-true
          # "Error Code if IMU not there"
          n143 = for {
            N: 22 -> [_]
            tunnel: u8 85 ("Data To Send 2") -> [w415]
            tunnel: w392 -> [w413] mode=indexing
            tunnel: w397 -> [w414]
            tunnel: [w408] -> w394
            tunnel: [w411] -> w386
            i -> [w416]
            n144 = Build Array(w413) -> (w412:u8[])
            n145 = Add(x=w415, y=w416) -> (x+y=w417:i32)
            n146 = call <vilib>:"WPI_I2CWrite.vi"("I2CDataToSend"=w412, "I2CRegister"=w417, "I2CDevRef"=w414) -> ("error out"=w410:errorcluster, "I2CDevRef"=w409:T2)  [unwired: 7 in]
            n147 = Bundle By Name(cluster=w409, "DevStatus"=w410) -> (w408:T2)
            n148 = Unbundle By Name(w410) -> ("code"=w411:i32)
          }
          n149 = Greater Or Equal?(x=w383, y=50) -> (x >= y?=w381:bool)
          n150 = for {
            N: 22 -> [_]
            tunnel: u8 85 ("Data To Send 2") -> [w404]
            tunnel: [w403] -> w393 mode=concatenating
            tunnel: w394 -> [w402]
            tunnel: [w401] -> w391
            i -> [w400]
            n151 = Add(x=w404, y=w400) -> (x+y=w405:i32)
            n152 = Build Array(w405) -> (w406:i32[])
            n153 = call <vilib>:"WPI_I2CRead.vi"("I2CBytesToRead"=u8 1, "I2CRegister"=w406, "I2CDevRef"=w402) -> ("Data Out"=w403:u8[], "I2CDevRef"=w401:T2)  [unwired: 6 in, 1 out]
          }
          n154 = Equal?(x=w386, y=-1) -> (x = y?=w384:bool)
          n155 = Equal?(x=w393, y=w392) -> (x = y?=w390:bool[])
          n156 = And Array Elements(Boolean array=w390) -> (logical AND=w388:bool)
          n157 = Compound Arithmetic op=OR(w388, w384, w381) -> (w387:bool)
          n158 = Wait (ms)(milliseconds to wait=u32 50) -> ()  [unwired: 1 out]
          "Restore Cal ct" <- w383
        }
        "Odd" <- w342
        n159 = Or(x=w339, y=w337) -> (x .or. y?=w338:bool)
        n160 = Build Array(w350) -> (w360:T10)
        n161 = call <vilib>:"WPI_I2CWrite.vi"("I2CDataToSend"=w360, "I2CRegister"=u8 61 ("Data To Send hex 2"), "I2CDevRef"=w351) -> ("I2CDevRef"=w349:T2)  [unwired: 7 in, 1 out]
        n162 = Select(t=Setup_State."Reset", s=w342, f=Setup_State."Cal Status") -> (s? t:f=w341:T7)
      }
      frame "Cal Status" {
        # "Poll the Cal_Status Register to indicate what the IMU reports regarding the calibration.\nContinue to update indicator for a set number of iterations to allow internal IMU Algo time to settle\nensuring IMU is ready for use once the IMUOpen operation has completed."
        n163 = while {
          tunnel: w423 -> [w435]
          tunnel: [w424] -> w420
          i -> [w434]
          stop <- w432 stop-if-true
          n164 = Build Array(u8 53 ("Data To Send")) -> (w436:u8[])
          n165 = call <vilib>:"WPI_I2CRead.vi"("I2CBytesToRead"=u8 1, "I2CRegister"=w436, "I2CDevRef"=w435) -> ("Data Out"=w447:u8[], "I2CDevRef"=w424:T2)  [unwired: 6 in, 1 out]
          n166 = Greater Or Equal?(x=w434, y="Status delay") -> (x >= y?=w432:bool)
          n167 = Index Array(array=w447) -> (element=w446:u8)  [unwired: 1 in]
          n168 = Number To Boolean Array(number=w446) -> (Boolean array=w445:bool[])
          n169 = Index Array(array=w445) -> (element #1=w439:bool, element #2=w440:bool, element #3=w426:bool, element #4=w448:bool, element #5=w441:bool, element #6=w442:bool, element #7=w443:bool, element #8=w444:bool)  [unwired: 8 in]
          n170 = Wait (ms)(milliseconds to wait=u32 2 ("pre-cal wait")) -> ()  [unwired: 1 out]
          n171 = call <userlib>:"Status.vi"("Big"=w440, "Little"=w439) -> ("Cluster"=w431:T11)  [unwired: 2 in]
          n172 = call <userlib>:"Status.vi"("Big"=w448, "Little"=w426) -> ("Cluster"=w430:T11)  [unwired: 2 in]
          n173 = call <userlib>:"Status.vi"("Big"=w442, "Little"=w441) -> ("Cluster"=w429:T11)  [unwired: 2 in]
          n174 = call <userlib>:"Status.vi"("Big"=w444, "Little"=w443) -> ("Cluster"=w428:T11)  [unwired: 2 in]
          n175 = Bundle("Cluster"=w431, "Cluster"=w430, "Cluster"=w429, "Cluster"=w428) -> (→"Cal Status @ Open":T4)  [unwired: 1 in]
        }
      }
      frame "Idle" {
        n176 = case shown="True" w457 {
          tunnel: [TRUE w462] -> w456
          tunnel: w455 -> [_ w459]
          frame False {
          }
          frame True {
            w465 = "\r\n"
            n177 = Concatenate Strings(w465, w465) -> (w461:string)
            n178 = Concatenate Strings("Your BNO055 calibration constants\nare stored in this file:" ("message"), w461, w459, w461, "Click OK when you have recorded the filename,\nthen stop the code, set Calibrate? to FALSE,\nand provide this filename to the\nIMUOrientOpen subVI \"Stored Cal File\" terminal." ("string"), w461, "When you next run IMUOrientOpen,\nthese calibration constants will be\nautomatically loaded and the IMU\nwill be ready for use upon startup." ("string"), w461, "The RoboBees Team 836 ... Orient to STEM!" ("string")) -> (w467:string)
            n179 = feedback #3(FALSE ("true")) -> (w469:bool)
            n180 = case shown="False" w469 {
              selector: w469 -> [_ w472]
              tunnel: [w471 w472] -> w462
              tunnel: w467 -> [w470 _]
              frame False {
                n181 = One Button Dialog(message=w470) -> (true=w471:bool)  [unwired: 1 in]
              }
              frame True {
              }
            }
            n182 = feedback-in #3(w462) -> ()
          }
        }
        n183 = Bundle By Name(cluster=w453, "DevStatus.status"=w451) -> (w452:T2)
      }
    }
    n184 = Bundle By Name(cluster=T1 {"I2CDevRef"={"DevStatus"={"status"=FALSE, "code"=0, "source"=""}, "Device Address"=0, "Handle"=0, "I2C Bus"=enum."Invalid"}, "Valid Cal File?"=FALSE} ("IMU Dev Ref"), "I2CDevRef"=w22, "Valid Cal File?"=w20) -> (w21:T1)
    "Setup ct" <- w39
    "Setup State" <- w28
  }
  "Bad Result" <- w13
  "Fatal Result" <- w9
  "error out" <- w3
  "IMU Dev Ref" <- w2
